vi "subAddDependencies.vi"(7 "Project path":path, 8 "error in (no error)":errorcluster, 9 "Dependencies":string[](array[string]), 10 "Name":string, 11 "SolutionBuilder in":refnum<class "SolutionBuilder.lvclass">) -> (0 "error out":errorcluster, 3 "SolutionBuilder out":refnum<class "SolutionBuilder.lvclass">)   [LabVIEW 2020, in "SolutionBuilder.lvlib" / "SolutionBuilder.lvclass"]
uses:
  SolutionBuilder.lvclass
  SolutionBuilder.lvclass/SolutionBuilder.ctl
  ProjectItem/ProjectItem.lvclass
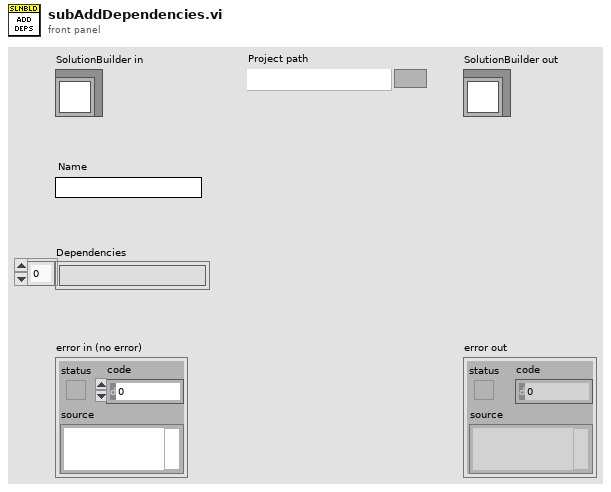
[diagram p1: front panel]
types:
  T1 = typedef "SolutionBuilder.lvlib/SolutionBuilder.lvclass/ProjectItemMap.ctl" = map{path, refnum<class "ProjectItem.lvclass">[]}
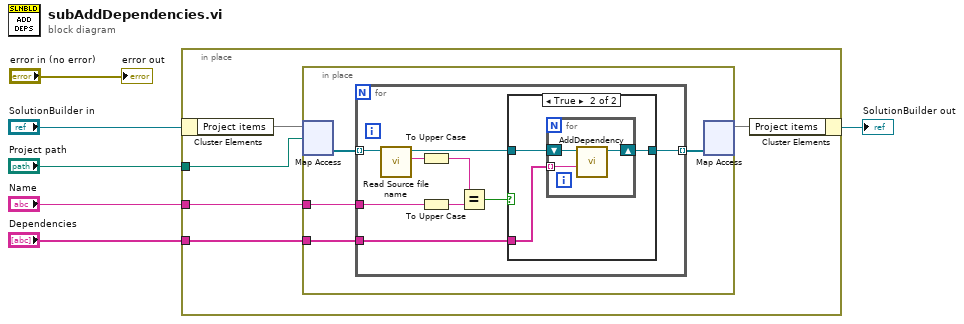
[diagram p0: block diagram]
diagram:
  n1 = in-place {
    in-place-border: "Project path" -> [w10]
    in-place-border: "Name" -> [w8]
    in-place-border: "Dependencies" -> [w7]
    n2 = in-place-cluster #1("SolutionBuilder in") -> ("Project items"=w11:T1)
    n3 = in-place {
      in-place-border: w8 -> [w14]
      in-place-border: w7 -> [w12]
      n4 = in-place-map #2(w11, w10) -> (w15:refnum<class "ProjectItem.lvclass">[])  [unwired: 1 in, 1 out]
      n5 = for {
        tunnel: w15 -> [w24] mode=indexing
        tunnel: w14 -> [w20]
        tunnel: [w17] -> w13 mode=indexing
        tunnel: w12 -> [w16]
        n6 = call-dynamic "Read Source file name.vi"("ProjectItem in"=w24) -> ("Source file name"=w23:string, "ProjectItem out"=w19:refnum<class "ProjectItem.lvclass">)  [unwired: 9 in]
        n7 = To Upper Case(1:w23) -> (0:w22:string)
        n8 = To Upper Case(1:w20) -> (0:w21:string)
        n9 = Equal?(x=w22, y=w21) -> (x = y?=w18:bool)
        n10 = case shown="True" w18 {
          tunnel: w19 -> [w25 w28]
          tunnel: [w25 w27] -> w17
          tunnel: w16 -> [_ w26]
          frame False {
          }
          frame True {
            n11 = for {
              shift-right: [w30] -> w27
              shift-left: w28 -> [w31]
              tunnel: w26 -> [w29] mode=indexing
              n12 = call-dynamic "AddDependency.vi"("Dependency"=w29, "ProjectItem in"=w31) -> ("ProjectItem out"=w30:refnum<class "ProjectItem.lvclass">)  [unwired: 8 in, 1 out]
            }
          }
        }
      }
      n13 = in-place-map #2(w13) -> (w9:T1)  [unwired: 1 in, 2 out]
    }
    n14 = in-place-cluster #1("Project items"=w9) -> (→"SolutionBuilder out":refnum<class "SolutionBuilder.lvclass">)
  }
  "error out" <- "error in (no error)"
